vi "day to time.vi"(2 "Time offset":timestamp, 3 "day":i32) -> (0 "day in absolute time":timestamp, 1 "day in seconds":dbl)   [LabVIEW 2019]
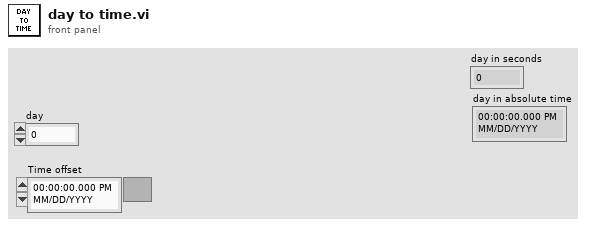
[diagram p1: front panel]
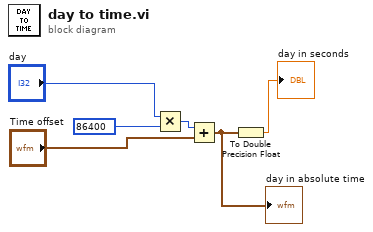
[diagram p0: block diagram]
diagram:
  n1 = Multiply(x="day", y=86400 ("Numeric")) -> (x*y=w6:i32)
  n2 = Add(x=w6, y="Time offset") -> (x+y=w4:timestamp)
  "day in absolute time" <- w4
  n3 = To Double Precision Float(number=w4) -> (double precision float=→"day in seconds":dbl)
